vi "Day 2.2 - .vi"(11 "input":string[](array[string])) -> (3 "ouptut part 2":u64)   [LabVIEW 2021]
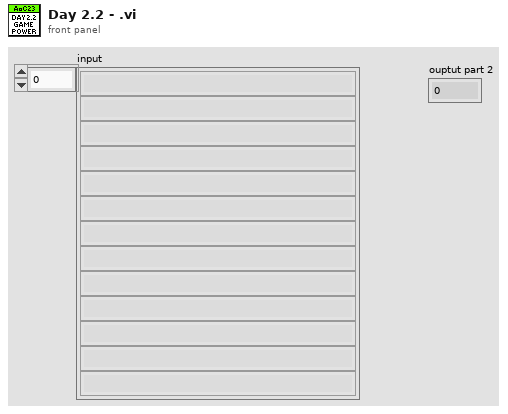
[diagram p1: front panel]
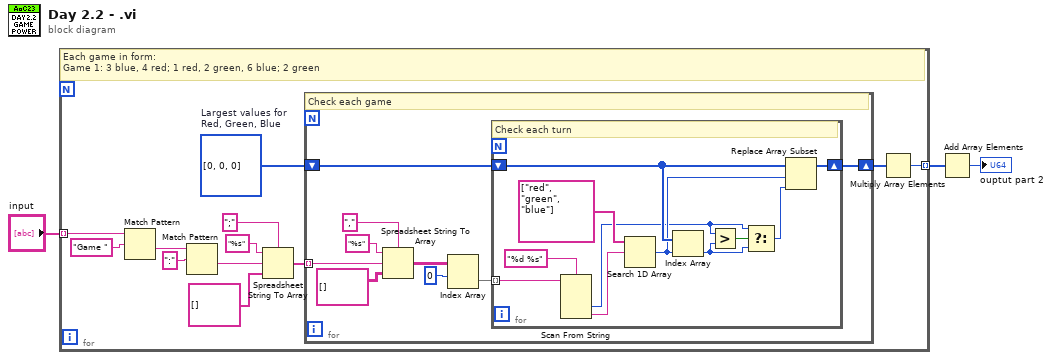
[diagram p0: block diagram]
diagram:
  n1 = for {
    tunnel: "input" -> [w12] mode=indexing
    tunnel: [w4] -> w1 mode=indexing
    w6 = i32[] [0, 0, 0]  # Largest values for Red, Green, Blue
    # "Each game in form:\nGame 1: 3 blue, 4 red; 1 red, 2 green, 6 blue; 2 green"
    n2 = Match Pattern(string=w12, regular expression="Game ") -> (after substring=w10:string)  [unwired: 1 in, 3 out]
    n3 = Match Pattern(string=w10, regular expression=":") -> (after substring=w8:string)  [unwired: 1 in, 3 out]
    n4 = Spreadsheet String To Array(delimiter (Tab)=";", format string="%s", spreadsheet string=w8, array type (2D Dbl)=string[] []) -> (array=w7:string[])
    n5 = for {
      tunnel: w7 -> [w24] mode=indexing
      shift-right: [w16] -> w5
      shift-left: w6 -> [w17]
      # "Check each game"
      n6 = Spreadsheet String To Array(delimiter (Tab)=",", format string="%s", spreadsheet string=w24, array type (2D Dbl)=string[][] []) -> (array=w20:string[][])
      n7 = Index Array(array=w20, index (row)=0) -> (element=w18:string[])  [unwired: 1 in]
      n8 = for {
        tunnel: w18 -> [w34] mode=indexing
        shift-right: [w30] -> w16
        shift-left: w17 -> [w31]
        # "Check each turn"
        n9 = Scan From String(format string="%d %s", input string=w34) -> (output 1=w27:i32, output 2=w32:string)  [unwired: 4 in, 3 out]
        n10 = Search 1D Array(1D array=string[] ["red", "green", "blue"], element=w32) -> (index of element=w29:i32)  [unwired: 1 in]
        n11 = Index Array(array=w31, index=w29) -> (element=w26:i32)
        n12 = Greater?(x=w27, y=w26) -> (0:w28:bool)
        n13 = Select(t=w27, s=w28, f=w26) -> (s? t:f=w25:i32)
        n14 = Replace Array Subset(array=w31, new element=w25, index=w29) -> (w30:i32[])
      }
    }
    n15 = Multiply Array Elements(1:w5) -> (0:w4:i32)
  }
  n16 = Add Array Elements(numeric array=w1) -> (sum=→"ouptut part 2":i32)
